vi "move_thru_motion_list.vi"(4 "error in (no error)":errorcluster, 5 "py interface file":path, 6 "Request data":variant, 7 "Python session in":refnum<k35>) -> (0 "error out":errorcluster, 2 "Response data":variant, 3 "Python session out":refnum<k35>)   [LabVIEW 2022 SP3]
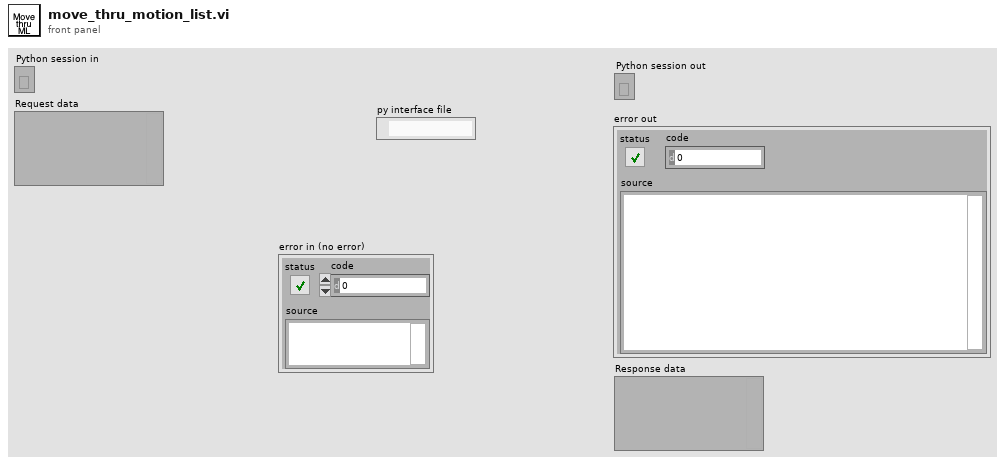
[diagram p1: front panel]
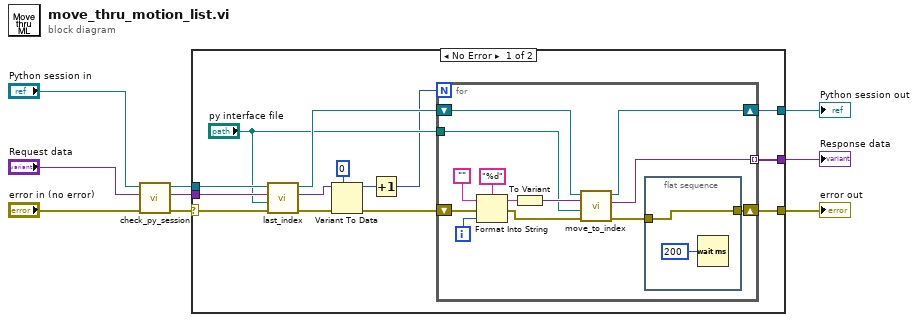
[diagram p0: block diagram]
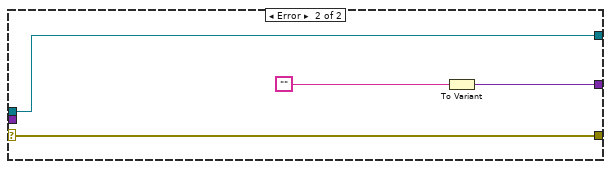
[diagram p2: hidden frame]
diagram:
  n1 = call "check_py_session.vi"("error in"="error in (no error)", "Request data"="Request data", "Python session in"="Python session in") -> ("error out"=w5:errorcluster, "Response data"=w6:variant, "Python session out"=w2:refnum<k35>)  [unwired: 2 in]
  n2 = case shown="No Error" w5 {
    selector: w5 -> [w22 w42]
    tunnel: w6 -> [w19 _]
    tunnel: [w16 w42] -> w4
    tunnel: [w15 w40] -> w3
    tunnel: w2 -> [w18 w39]
    tunnel: [w14 w39] -> w1
    frame No Error {
      n3 = call "last_index.vi"("error in (no error)"=w22, "py interface file"="py interface file", "Request data"=w19, "Python session in"=w18) -> ("error out"=w21:errorcluster, "Response data"=w20:variant, "Python session out"=w13:refnum<k35>)  [unwired: 1 in]
      n4 = Variant To Data(error in=w21, type=0, Variant=w20) -> (data=w11:i32, error out=w17:errorcluster)
      n5 = Increment(x=w11) -> (x+1=w10:i32)
      n6 = for {
        N: w10 -> [_]
        shift-right: [w24] -> w16
        shift-left: w17 -> [w35]
        tunnel: [w30] -> w15 mode=indexing
        shift-right: [w29] -> w14
        shift-left: w13 -> [w28]
        tunnel: "py interface file" -> [w26]
        i -> [w34]
        n7 = Format Into String(format string="%d", initial string="", error in=w35, w34) -> (resulting string=w32:string, error out=w31:errorcluster)
        n8 = To Variant(anything=w32) -> (Variant=w27:variant)
        n9 = call "move_to_index.vi"("error in (no error)"=w31, "py interface file"=w26, "Request data"=w27, "Python session in"=w28) -> ("error out"=w25:errorcluster, "Response data"=w30:variant, "Python session out"=w29:refnum<k35>)  [unwired: 1 in]
        n10 = flat-sequence {
          tunnel: w25 -> [w38]
          tunnel: [w38] -> w24
          frame #0 {
            n11 = Wait (ms)(milliseconds to wait=u32 200) -> ()  [unwired: 1 out]
          }
        }
      }
    }
    frame Error {
      n12 = To Variant(anything="") -> (Variant=w40:variant)
    }
  }
  "error out" <- w4
  "Python session out" <- w1
  "Response data" <- w3
